vi "Image Index - FGV.vi"(8 "Error In":errorcluster, 10 "set image index":i16, 11 "Actions":T1=enum."Set") -> (0 "Error Out":errorcluster, 3 "image index":i16)   [LabVIEW 2017]
uses:
  Controls/FGV Actions.ctl
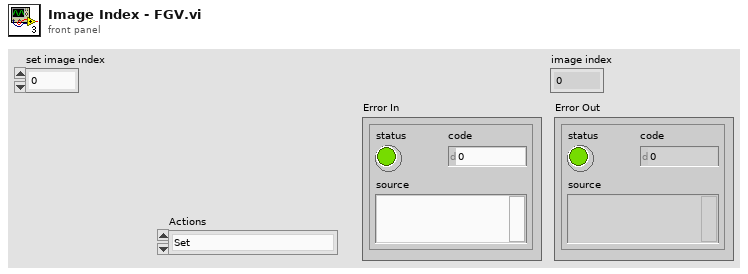
[diagram p1: front panel]
types:
  T1 = typedef "FGV Actions.ctl" = enum16{"Init", "Set", "Get", "Clear"}
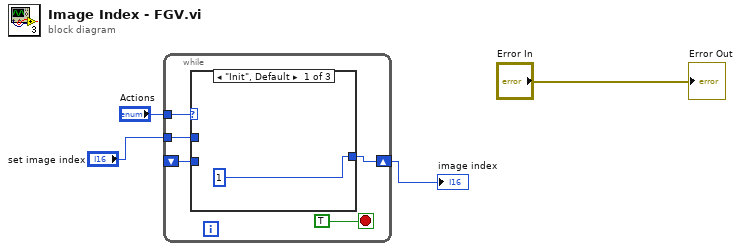
[diagram p0: block diagram]
diagram:
  n1 = while {
    tunnel: "Actions" -> [w8]
    tunnel: "set image index" -> [w5]
    shift-right: [w7] -> w1
    shift-left: _ -> [w6]
    stop <- TRUE stop-if-true
    n2 = case shown="\"Init\", Default" w8 {
      tunnel: w5 -> [_ w11 _]
      tunnel: [i16 1 w11 w12] -> w7
      tunnel: w6 -> [_ _ w12]
      frame "Init", Default {
      }
      frame "Set" {
      }
      frame "Get" {
      }
    }
  }
  "image index" <- w1
  "Error Out" <- "Error In"
